vi "Logging Message Loop.vi"(8 "error in (no error)":errorcluster, 10 "Queue B -TDMS Raw":refnum<queue>, 11 "Message Queues":T1) -> (0 "error out":errorcluster)   [LabVIEW 2026, in "Logging.lvlib"]
doc: "The message loop subVI to handle messages pertaining to logging data."
uses:
  Logging.lvlib
  support/Architecture/Message Queue/All Message Queues.ctl
  support/Architecture/Message Queue/Message Cluster.ctl
  Logging Configuration.ctl
  Logging State.ctl
  support/Architecture/Message Queue/Enqueue Message (Single).vi
  <vilib>/Utility/error.llb/Error Cluster From Error Code.vi
  <vilib>/ErrorRing/Error Ring.xnode
  support/Architecture/Message Queue/Message Queue.lvlib
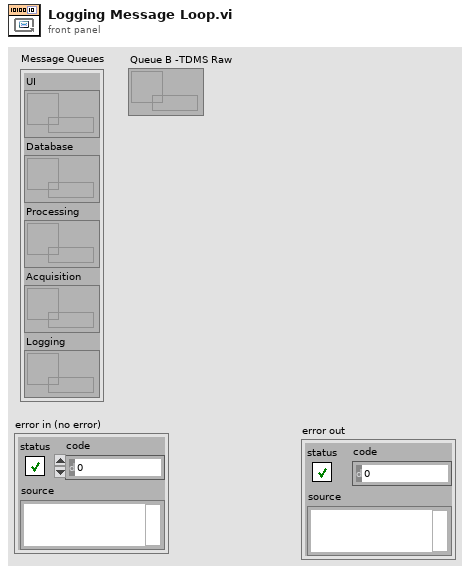
[diagram p1: front panel]
types:
  T1 = typedef "Message Queue.lvlib/All Message Queues.ctl" = cluster{"UI":refnum<queue>, "Database":refnum<queue>, "Processing":refnum<queue>, "Acquisition":refnum<queue>, "Logging":refnum<queue>}
  T2 = enum16{"open", "open or create", "create or replace", "create", "open (read-only)"}
  T3 = typedef "Logging.lvlib/Logging State.ctl" = enum16{"Idle", "Logging"}
  T4 = typedef "Logging.lvlib/Logging Configuration.ctl" = cluster{"Log File Base Path":path, "TDMS File Reference":refnum<k34>}
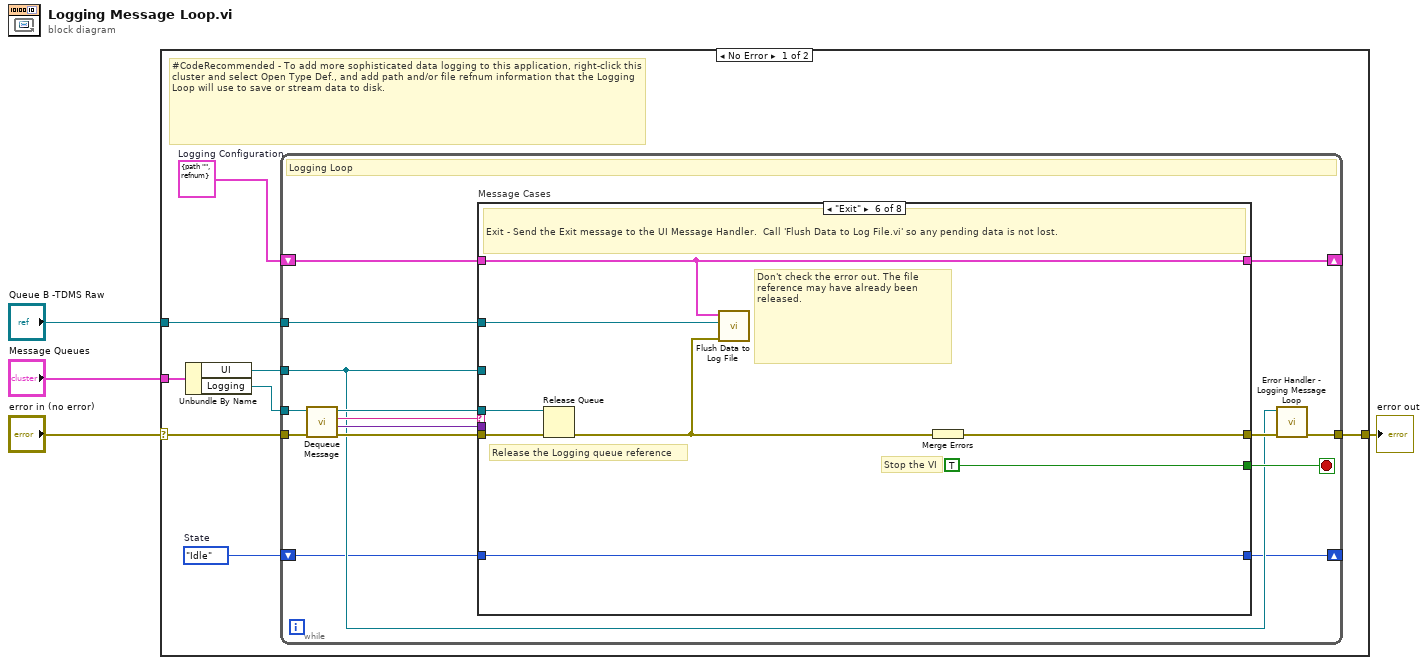
[diagram p0: block diagram]
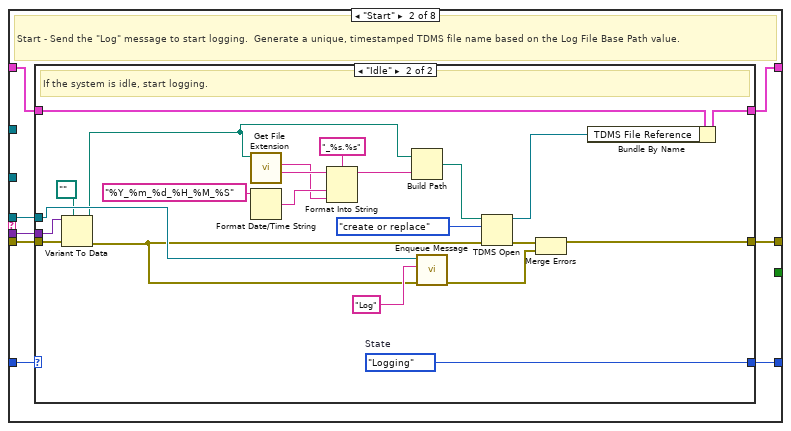
[diagram p3: hidden frame]
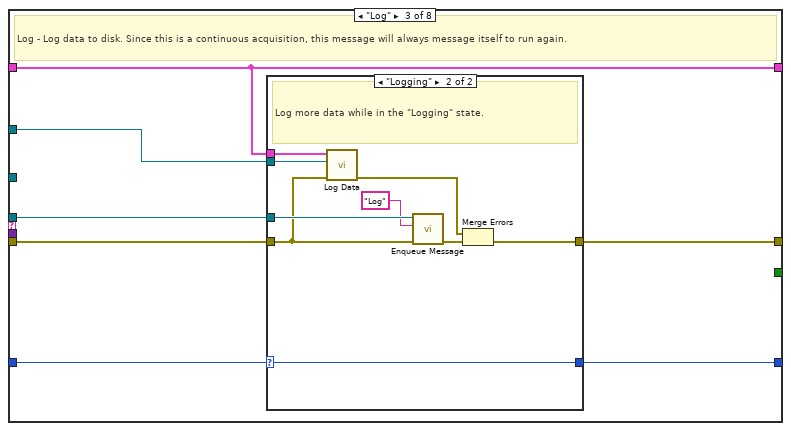
[diagram p5: hidden frame]
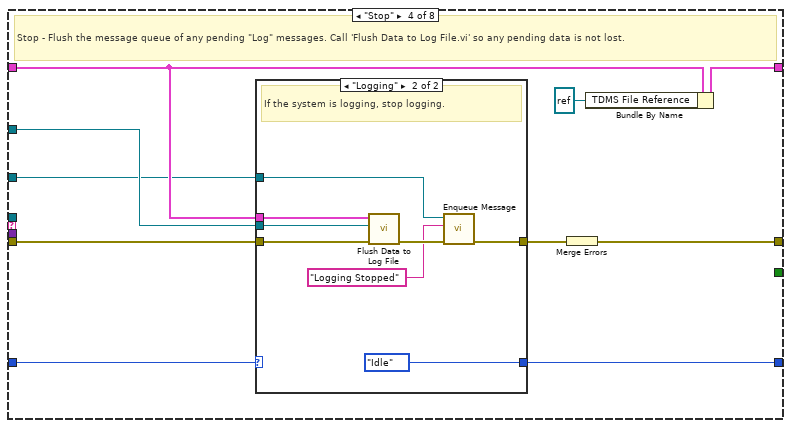
[diagram p7: hidden frame]
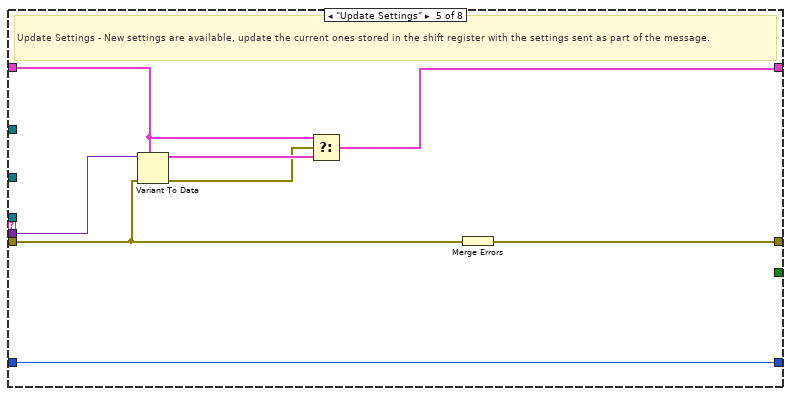
[diagram p9: hidden frame]
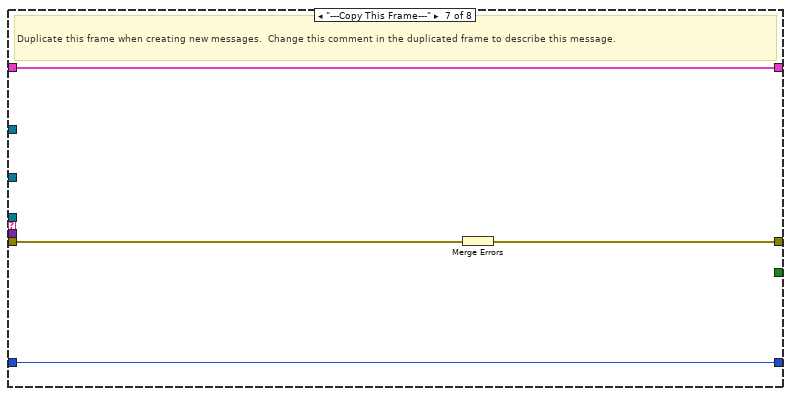
[diagram p10: hidden frame]
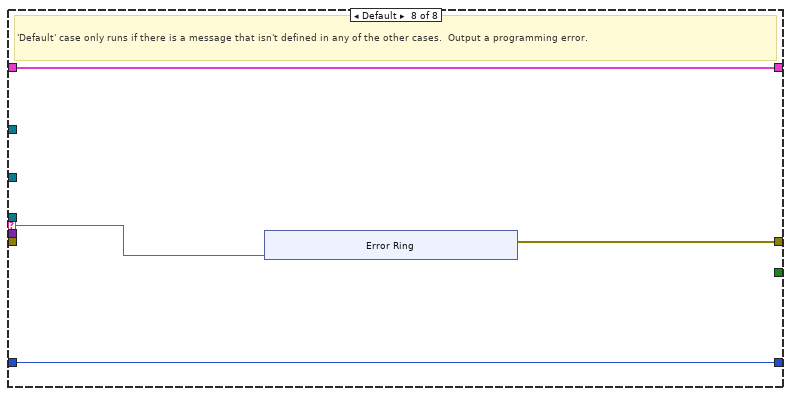
[diagram p11: hidden frame]
diagram:
  n1 = case shown="No Error" "error in (no error)" {
    selector: "error in (no error)" -> [w8 w133]
    tunnel: "Message Queues" -> [w12 _]
    tunnel: [w10 w133] -> w3
    tunnel: "Queue B -TDMS Raw" -> [w7 _]
    frame No Error {
      w5 = Logging_State."Idle"  # State
      w9 = T4 {"Log File Base Path"=path "", "TDMS File Reference"=refnum}  # Logging Configuration
      # "#CodeRecommended - To add more sophisticated data logging to this application, right-click this cluster and select Open Type Def., and add path and/or file refnum information that the Logging Loop will use to save or stream data to disk."
      n2 = Unbundle By Name(w12) -> ("UI"=w6:refnum<queue>, "Logging"=w11:refnum<queue>)
      n3 = while {
        tunnel: w11 -> [w19]
        shift-right: [w26] -> _
        shift-left: w9 -> [w27]
        tunnel: w6 -> [w15]
        tunnel: w7 -> [w18]
        tunnel: w8 -> [w24]
        tunnel: [w17] -> w10
        shift-right: [w13] -> _
        shift-left: w5 -> [w14]
        stop <- w25 stop-if-true
        # "Logging Loop"
        n4 = call "Dequeue Message.vi"("error in (no error)"=w24, "Message Queue"=w19) -> ("error out"=w23:errorcluster, "Message Data"=w21:variant, "Message"=w22:string, "dup Message Queue"=w20:refnum<queue>)  [unwired: 6 in]
        n5 = case "Message Cases" shown="\"Exit\"" w22 {
          selector: w22 -> [_ _ _ _ _ _ _ w123]
          tunnel: w20 -> [_ w37 w69 _ _ w114 _ _]
          tunnel: w23 -> [w29 w36 w67 w85 w103 w115 w121 _]
          tunnel: [w29 w38 w70 w91 w109 w116 w119 w124] -> w16
          tunnel: w27 -> [w30 w35 w66 w86 w107 w110 w120 w125]
          tunnel: [w30 w34 w66 w89 w104 w110 w120 w125] -> w26
          tunnel: [_ _ _ _ _ TRUE _ _] -> w25
          tunnel: w21 -> [_ w33 _ _ w108 _ _ _]
          tunnel: w15 -> [_ _ _ w84 _ _ _ _]
          tunnel: w18 -> [_ _ w68 w87 _ w112 _ _]
          tunnel: w14 -> [w28 w32 w65 w83 w102 w111 w118 w122]
          tunnel: [w28 w31 w64 w82 w102 w111 w118 w122] -> w13
          frame "Initialize" {
            # "Initialize - gets called when first launched. Currently a no-op."
          }
          frame "Start" {
            # "Start - Send the \"Log\" message to start logging.  Generate a unique, timestamped TDMS file name based on the Log File Base Path value."
            n6 = case shown="\"Idle\"" w32 {
              selector: w32 -> [w39 _]
              tunnel: [w40 w49] -> w38
              tunnel: w37 -> [_ w46]
              tunnel: w36 -> [w40 w48]
              tunnel: w35 -> [w41 w50]
              tunnel: [w41 w51] -> w34
              tunnel: w33 -> [_ w47]
              tunnel: [w39 w42] -> w31
              frame "Logging" {
                # "The system is already logging. Ignore the \"Start\" message."
              }
              frame "Idle" {
                w42 = Logging_State."Logging"  # State
                # "If the system is idle, start logging."
                n7 = Variant To Data(error in=w48, type=path "", Variant=w47) -> (data=w43:path, error out=w45:errorcluster)
                n8 = call <vilib>:"Get File Extension.vi"("file"=w43) -> ("filename without extension"=w61:string, "lowercase file extension"=w58:string)  [unwired: 6 in, 3 out]
                n9 = Format Date/Time String(time format string (%c)="%Y_%m_%d_%H_%M_%S") -> (date/time string=w59:string)  [unwired: 2 in]
                n10 = Format Into String(format string="_%s.%s", initial string=w61, w59, w58) -> (resulting string=w57:string)  [unwired: 1 in, 1 out]
                n11 = Build Path(base path=w43, name or relative path=w57) -> (appended path=w56:path)
                n12 = call-poly "Enqueue Message.vi"("error in (no error)"=w45, "Message"="Log", "Message Queue"=w46) -> ("error out"=w54:errorcluster)  [unwired: 7 in, 1 out]
                n13 = TDMS Open(8:w45, 10:T2."create or replace" ("operation (0:open)"), 11:w56) -> (0:w55:errorcluster, 3:w52:refnum<k34>)  [unwired: 4 in]
                n14 = Merge Errors(w55, w54) -> (w49:errorcluster)
                n15 = Bundle By Name(cluster=w50, "TDMS File Reference"=w52) -> (w51:T4)
              }
            }
          }
          frame "Log" {
            # "Log - Log data to disk. Since this is a continuous acquisition, this message will always message itself to run again."
            n16 = case shown="\"Logging\"" w65 {
              selector: w65 -> [w72 w74]
              tunnel: [w71 w81] -> w70
              tunnel: w69 -> [_ w79]
              tunnel: w68 -> [_ w78]
              tunnel: w67 -> [w71 w73]
              tunnel: w66 -> [_ w75]
              tunnel: [w72 w74] -> w64
              frame "Idle" {
                # "Ignore \"Log\" messages when the logging is idle."
              }
              frame "Logging" {
                # "Log more data while in the \"Logging\" state."
                n17 = call "Log Data.vi"("error in (no error)"=w73, "Queue B -TDMS Raw"=w78, "Logging Configuration"=w75) -> ("error out"=w77:errorcluster)  [unwired: 8 in]
                n18 = call-poly "Enqueue Message.vi"("error in (no error)"=w73, "Message"="Log", "Message Queue"=w79) -> ("error out"=w80:errorcluster)  [unwired: 7 in, 1 out]
                n19 = Merge Errors(w77, w80) -> (w81:errorcluster)
              }
            }
          }
          frame "Stop" {
            # "Stop - Flush the message queue of any pending \"Log\" messages. Call 'Flush Data to Log File.vi' so any pending data is not lost."
            n20 = case shown="\"Logging\"" w83 {
              selector: w83 -> [w92 _]
              tunnel: [w93 w98] -> w90
              tunnel: w87 -> [_ w94]
              tunnel: w86 -> [_ w100]
              tunnel: w85 -> [w93 w99]
              tunnel: w84 -> [_ w97]
              tunnel: [w92 Logging_State."Idle" ("State")] -> w82
              frame "Idle" {
                # "The system is already idle. Ignore the \"Stop\" message."
              }
              frame "Logging" {
                # "If the system is logging, stop logging."
                n21 = call "Flush Data to Log File.vi"("error in (no error)"=w99, "Data Queue"=w94, "Logging Configuration"=w100) -> ("error out"=w101:errorcluster)  [unwired: 8 in]
                n22 = call-poly "Enqueue Message.vi"("error in (no error)"=w101, "Message"="Logging Stopped", "Message Queue"=w97) -> ("error out"=w98:errorcluster)  [unwired: 7 in, 1 out]
              }
            }
            n23 = Merge Errors(w90) -> (w91:errorcluster)
            n24 = Bundle By Name(cluster=w86, "TDMS File Reference"=refnum<k34> refnum) -> (w89:T4)
          }
          frame "Update Settings" {
            # "Update Settings - New settings are available, update the current ones stored in the shift register with the settings sent as part of the message."
            n25 = Variant To Data(error in=w103, type=w107, Variant=w108) -> (data=w106:T4, error out=w105:errorcluster)
            n26 = Select(t=w107, s=w105, f=w106) -> (s? t:f=w104:T4)
            n27 = Merge Errors(w103) -> (w109:errorcluster)
          }
          frame "Exit" {
            # "Don't check the error out. The file reference may have already been released."
            # "Release the Logging queue reference"
            # "Stop the VI"
            # "Exit - Send the Exit message to the UI Message Handler.  Call 'Flush Data to Log File.vi' so any pending data is not lost."
            n28 = Release Queue(queue=w114, error in (no error)=w115) -> (error out=w113:errorcluster)  [unwired: 1 in, 2 out]
            n29 = call "Flush Data to Log File.vi"("error in (no error)"=w113, "Data Queue"=w112, "Logging Configuration"=w110) -> ()  [unwired: 8 in, 1 out]
            n30 = Merge Errors(w113) -> (w116:errorcluster)
          }
          frame "---Copy This Frame---" {
            # "Duplicate this frame when creating new messages.  Change this comment in the duplicated frame to describe this message."
            n31 = Merge Errors(w121) -> (w119:errorcluster)
          }
          frame Default {
            # "'Default' case only runs if there is a message that isn't defined in any of the other cases.  Output a programming error."
            n32 = xnode "Error Ring"("parameter 0"=w123) -> ("error out"=w124:errorcluster)
          }
        }
        n33 = call "Error Handler - Logging Message Loop.vi"("error in (no error)"=w16, "Message Queue"=w15) -> ("dup error in"=w17:errorcluster)  [unwired: 8 in, 1 out]
      }
    }
    frame Error {
    }
  }
  "error out" <- w3
